vi "Cond Attr Get Process.vi"(8 "error in (no error)":errorcluster, 11 "Cond Attr in":T2) -> (0 "error out":errorcluster, 2 "process":T1, 3 "Cond Attr out":T2)   [LabVIEW 2013, in "Linux RT IPC.lvlib" / "POSIX Threads.lvlib" / "Cond Attr.lvclass"]
doc: "Calls pthread_condattr_getpshared() on the pthread cond attribute object encapsulated by Cond Attr.\n\nThis VI returns the process scope for the conditional variable.\n\nRefer to online POSIX documentation for more information."
uses:
  Cond Attr.lvclass
  Controls/reference.ctl
  Controls/Public/C Enums/pthread_process_shared.ctl
  POSIX Thread Object/POSIX Thread Object.lvclass/POSIX Thread Object.ctl
  POSIX Thread Object/Private VIs/libpthread path.vi
  POSIX Thread Object/Private VIs/get pthread error.vi
  POSIX Thread Object/POSIX Thread Object.lvclass
  POSIX Threads.lvlib
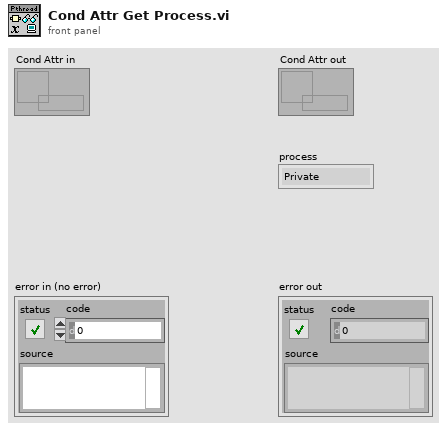
[diagram p1: front panel]
types:
  T1 = typedef "Linux RT IPC.lvlib/POSIX Threads.lvlib/pthread_process_shared.ctl" = enum16{"Private", "Shared"}
  T2 = typedef "Linux RT IPC.lvlib/POSIX Threads.lvlib/Cond Attr.lvclass/reference.ctl" = refnum<data-value>
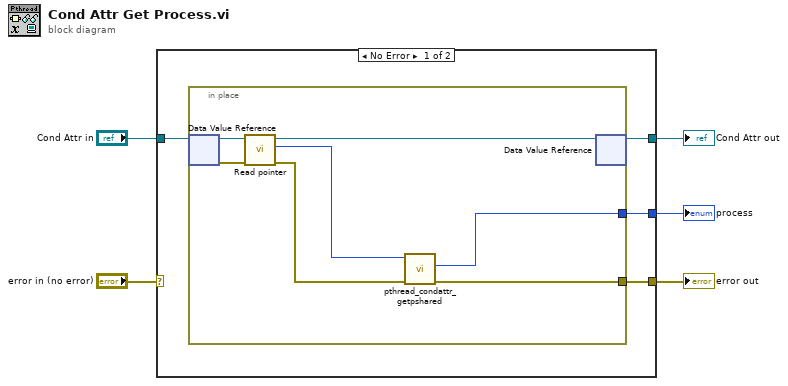
[diagram p0: block diagram]
diagram:
  n1 = case shown="No Error" "error in (no error)" {
    selector: "error in (no error)" -> [_ w18]
    tunnel: [w7 w18] -> w4
    tunnel: "Cond Attr in" -> [w9 w17]
    tunnel: [w8 w17] -> w2
    tunnel: [w6 _] -> w1
    frame No Error {
      n2 = in-place {
        in-place-border: [w12] -> w7
        in-place-border: [w10] -> w6
        n3 = in-place-dvr #1(w9) -> (w16:refnum<class "Cond Attr.lvclass">, w14:errorcluster)
        n4 = call "Read pointer.vi"("error in (no error)"=w14, "POSIX Thread Object in"=w16) -> ("error out"=w13:errorcluster, "pointer"=w11:u64, "POSIX Thread Object out"=w15:refnum<class "Cond Attr.lvclass">)  [unwired: 7 in]
        n5 = call "pthread_condattr_getpshared.vi"("error in (no error)"=w13, "cond attr ptr in"=w11) -> ("error out"=w12:errorcluster, "process shared"=w10:T1)  [unwired: 7 in, 1 out]
        n6 = in-place-dvr #1(w15) -> (w8:T2)  [unwired: 1 out]
      }
    }
    frame Error {
    }
  }
  "Cond Attr out" <- w2
  "error out" <- w4
  "process" <- w1
